vi "Param_Analysis_7_24b_JW.vi"(6 "Independant Variable":string, 7 "error in (no error)":errorcluster, 8 "Data Folder":path=path "D:/Userdata/Documents/Lab/8_26/diF-TES ADT 0_33pct cB_SAC-Shaker/data", 9 "Parameter String":string, 10 "Parameter Name":string, 11 "Stats Folder":path=path "D:/Userdata/Documents/Lab/8_26/diF-TES ADT 0_33pct cB_SAC-Shaker/data") -> (0 "Output File":path=path "D:/Userdata/Documents/Lab/8_26/diF-TES ADT 0_33pct cB_SAC-Shaker/data", 1 "error out":errorcluster, 2 "Output Array":string[][](array[string]), 3 "Variables":T1)   [LabVIEW 2012]
doc: "Stats Folder - Directory where the analysis is to be stored\n\nData Folder - Directory where the files to be analyzed are stored\n\nParameter Name - String to be used as the name of the outputed file for the analyzed paramters \n\nParameter String - String that should be identically equal to the name adjacent to the parameter to be analyzed in the data files\n\n\nOutput File - Directory where the analysis summary is located"
uses:
  <vilib>/Utility/file.llb/Read From Spreadsheet File (string).vi
  <vilib>/Utility/file.llb/Write To Spreadsheet File (string).vi
panel:
  out "Resulting Time Stamp":timestamp
  out "String":string
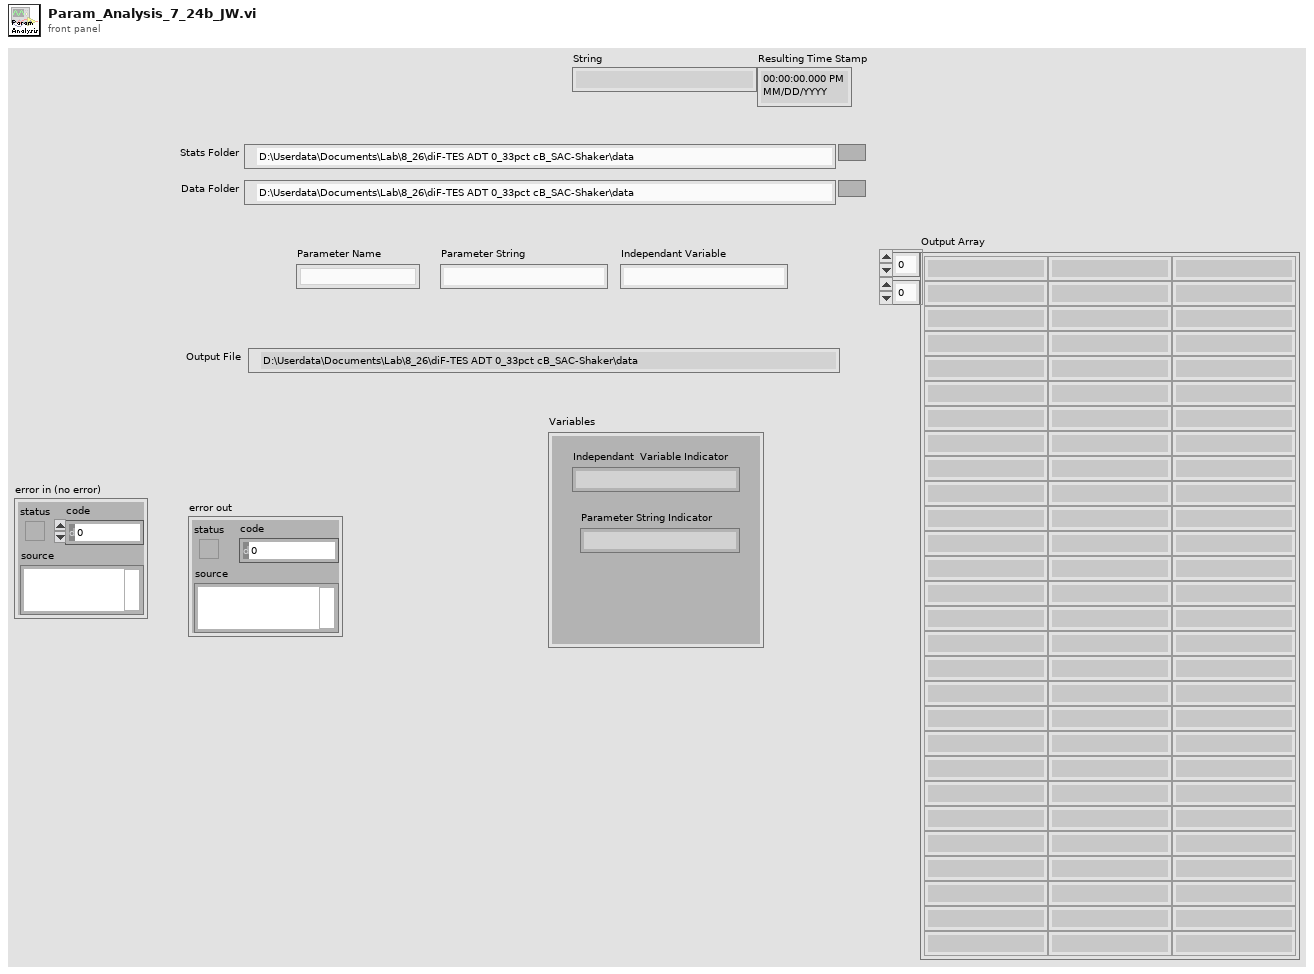
[diagram p1: front panel]
types:
  T1 = cluster{"Independant  Variable Indicator":string, "Parameter String Indicator":string}
  T2 = cluster{"Independant Variable":string, "Parameter String":string}
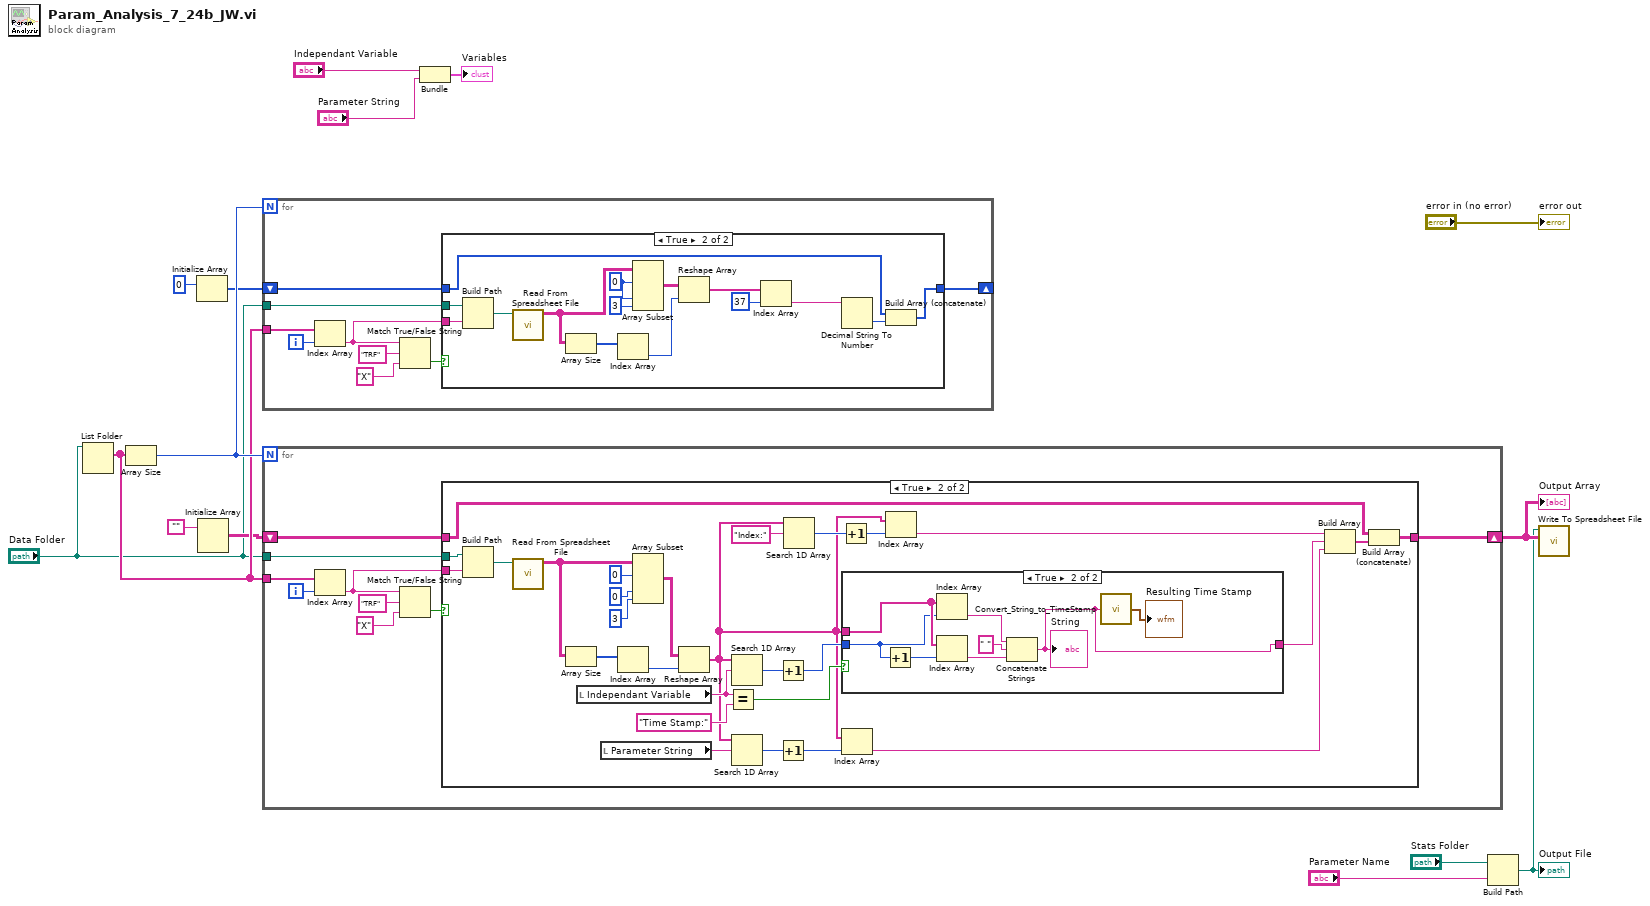
[diagram p0: block diagram]
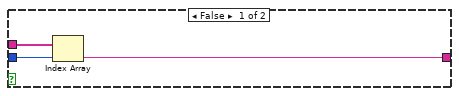
[diagram p3: hidden frame]
diagram:
  n1 = List Folder(path="Data Folder") -> (filenames=w14:string[])  [unwired: 3 in, 3 out]
  n2 = Array Size(array=w14) -> (size(s)=w15:i32)
  n3 = Initialize Array(0) -> (w12:i32[])  [unwired: 1 in]
  n4 = Initialize Array("") -> (w9:string[][])  [unwired: 2 in]
  n5 = for {
    N: w15 -> [_]
    tunnel: w14 -> [w24]
    tunnel: "Data Folder" -> [w22]
    shift-right: [w17] -> _
    shift-left: w12 -> [w16]
    i -> [w23]
    n6 = Index Array(array=w24, index=w23) -> (element=w21:string)
    n7 = Match True/False String(2:"X", 3:"TRF", 4:w21) -> (0:w19:bool)  [unwired: 1 out]
    n8 = case shown="True" w19 {
      tunnel: w22 -> [_ w40]
      tunnel: w21 -> [_ w32]
      tunnel: [w25 w31] -> w17
      tunnel: w16 -> [w25 w30]
      frame False {
      }
      frame True {
        w37 = 0
        n9 = Build Path(base path=w40, name or relative path=w32) -> (appended path=w39:path)
        n10 = call-poly <vilib>:"Read From Spreadsheet File.vi"("file path (dialog if empty)"=w39) -> ("all rows"=w35:string[][])  [unwired: 6 in, 4 out]
        n11 = Array Size(array=w35) -> (size(s)=w36:i32[])
        n12 = Index Array(array=w36) -> (element=w34:i32)  [unwired: 1 in]
        n13 = Array Subset(array=w35, index (row)=w37, index (col)=w37, length (col)=3) -> (w33:string[][])  [unwired: 1 in]
        n14 = Reshape Array(w33, w34) -> (w27:string[])
        n15 = Index Array(array=w27, index=37) -> (element=w29:string)
        n16 = Decimal String To Number(string=w29) -> (number=w28:i32)  [unwired: 2 in, 1 out]
        n17 = Build Array (concatenate)(w30, w28) -> (w31:i32[])
      }
    }
  }
  n18 = for {
    N: w15 -> [_]
    tunnel: w14 -> [w49]
    tunnel: "Data Folder" -> [w47]
    shift-right: [w42] -> w8
    shift-left: w9 -> [w41]
    i -> [w48]
    n19 = Index Array(array=w49, index=w48) -> (element=w46:string)
    n20 = Match True/False String(2:"X", 3:"TRF", 4:w46) -> (0:w44:bool)  [unwired: 1 out]
    n21 = case shown="True" w44 {
      tunnel: w47 -> [_ w78]
      tunnel: w46 -> [_ w71]
      tunnel: [w50 w67] -> w42
      tunnel: w41 -> [w50 w66]
      frame False {
      }
      frame True {
        n22 = Build Path(base path=w78, name or relative path=w71) -> (appended path=w77:path)
        n23 = call-poly <vilib>:"Read From Spreadsheet File.vi"("file path (dialog if empty)"=w77) -> ("all rows"=w60:string[][])  [unwired: 6 in, 4 out]
        n24 = Array Size(array=w60) -> (size(s)=w74:i32[])
        n25 = local read "Independant Variable"() -> (w55:string)
        n26 = local read "Parameter String"() -> (w57:string)
        n27 = Index Array(array=w74) -> (element=w73:i32)  [unwired: 1 in]
        n28 = Array Subset(array=w60, index (row)=0, index (col)=0, length (col)=3) -> (w72:string[][])  [unwired: 1 in]
        n29 = Reshape Array(w72, w73) -> (w52:string[])
        n30 = Equal?(x=w55, y="Time Stamp:") -> (x = y?=w54:bool)
        n31 = Search 1D Array(1D array=w52, element=w55) -> (index of element=w65:i32)  [unwired: 1 in]
        n32 = Search 1D Array(1D array=w52, element=w57) -> (index of element=w70:i32)  [unwired: 1 in]
        n33 = Increment(x=w65) -> (x+1=w53:i32)
        n34 = Increment(x=w70) -> (x+1=w69:i32)
        n35 = Search 1D Array(1D array=w52, element="Index:") -> (index of element=w63:i32)  [unwired: 1 in]
        n36 = Increment(x=w63) -> (x+1=w62:i32)
        n37 = case shown="True" w54 {
          tunnel: w53 -> [w80 w87]
          tunnel: w52 -> [w81 w89]
          tunnel: [w79 w83] -> w51
          frame False {
            n38 = Index Array(array=w81, index=w80) -> (element=w79:string)
          }
          frame True {
            n39 = Increment(x=w87) -> (x+1=w88:i32)
            n40 = Index Array(array=w89, index=w87) -> (element=w86:string)
            n41 = Index Array(array=w89, index=w88) -> (element=w85:string)
            n42 = Concatenate Strings(w86, " " ("string"), w85) -> (w83:string)
            "String" <- w83
            n43 = call "Convert_String_to_TimeStamp.vi"("date/time string"=w83) -> ("Resulting Time Stamp"=→"Resulting Time Stamp":timestamp)
          }
        }
        n44 = Index Array(array=w52, index=w69) -> (element=w58:string)
        n45 = Index Array(array=w52, index=w62) -> (element=w61:string)
        n46 = Build Array(w61, w51, w58) -> (w68:string[])
        n47 = Build Array (concatenate)(w66, w68) -> (w67:string[][])
      }
    }
  }
  "Output Array" <- w8
  n48 = Bundle("Independant Variable"="Independant Variable", "Parameter String"="Parameter String") -> (→"Variables":T2)  [unwired: 1 in]
  n49 = Build Path(base path="Stats Folder", name or relative path="Parameter Name") -> (appended path=w7:path)
  "Output File" <- w7
  n50 = call-poly <vilib>:"Write To Spreadsheet File.vi"("2D data"=w8, "file path (dialog if empty)"=w7) -> ()  [unwired: 6 in, 1 out]
  "error out" <- "error in (no error)"
